vi "DereferencingPointerToComplexStructUsingGetValueByPointer.vi"(8 "error in (no error)":errorcluster, 11 "Pointer":i64) -> (0 "error out":errorcluster, 3 "ComplexStruct Polygon":T1)   [LabVIEW 2009, in "LabVIEWWrapper_PassingDataSampleDLL.lvlib"]
uses:
  LabVIEWWrapper_PassingDataSampleDLL.lvlib
  CustomControlsForStructs/ComplexStruct Polygon.ctl
  <vilib>/Utility/importsl/GetValueByPointer/GetValueByPointer.xnode
  <vilib>/Utility/importsl/GetValueByPointer/datatype.ctl
  Program Files (x86)/National Instruments/LabVIEW 2009/resource/lvimptsl.dll
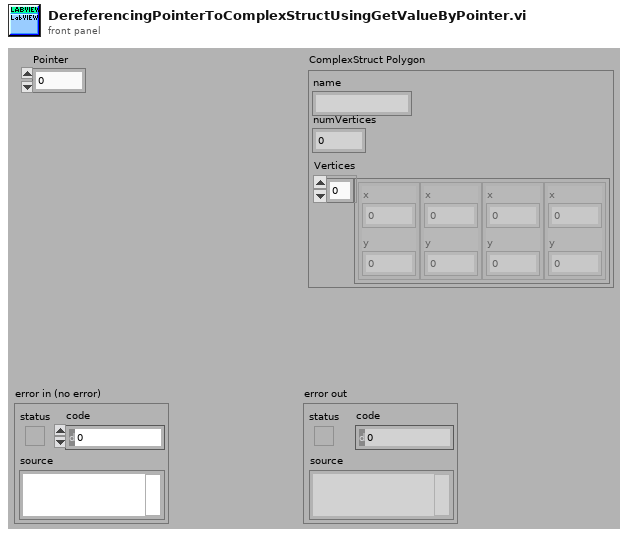
[diagram p1: front panel]
types:
  T1 = typedef "LabVIEWWrapper_PassingDataSampleDLL.lvlib/ComplexStruct Polygon.ctl" = cluster{"name":string, "numVertices":i32, "Vertices":cluster{"x":i32, "y":i32}[]}
  T2 = cluster{"Output":string, "Output":i32, cluster{"Output":i32, "Output":i32}[]}
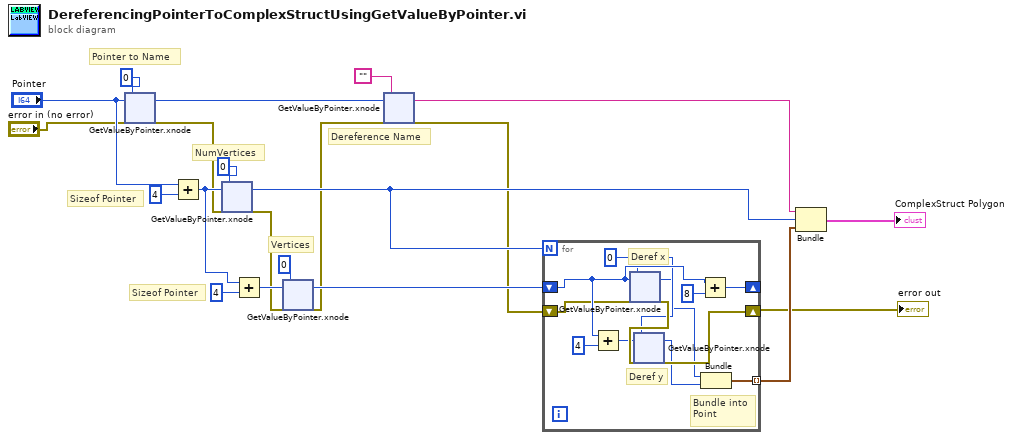
[diagram p0: block diagram]
diagram:
  # "Sizeof Pointer"
  # "Sizeof Pointer"
  # "Dereference Name"
  # "Vertices"
  # "NumVertices"
  # "Pointer to Name"
  n1 = xnode "GetValueByPointer.xnode"("Pointer"="Pointer", "InputType"=0, "ErrorIn"="error in (no error)") -> ("Output"=w20:i32, "ErrorOut"=w6:errorcluster)  [unwired: 1 in]
  n2 = Add(x="Pointer", y=i64 4) -> (x+y=w15:i64)
  n3 = xnode "GetValueByPointer.xnode"("Pointer"=w15, "InputType"=0, "ErrorIn"=w6) -> ("Output"=w9:i32, "ErrorOut"=w5:errorcluster)  [unwired: 1 in]
  n4 = Add(x=w15, y=i64 4) -> (x+y=w16:i64)
  n5 = xnode "GetValueByPointer.xnode"("Pointer"=w16, "InputType"=0, "ErrorIn"=w5) -> ("Output"=w14:i32, "ErrorOut"=w3:errorcluster)  [unwired: 1 in]
  n6 = xnode "GetValueByPointer.xnode"("Pointer"=w20, "InputType"="", "ErrorIn"=w3) -> ("Output"=w10:string, "ErrorOut"=w1:errorcluster)  [unwired: 1 in]
  n7 = for {
    N: w9 -> [_]
    shift-right: [w28] -> _
    shift-left: w14 -> [w29]
    shift-right: [w26] -> w4
    shift-left: w1 -> [w27]
    tunnel: [w22] -> w8 mode=indexing
    w25 = 0
    # "Deref y"
    # "Deref x"
    # "Bundle into\nPoint"
    n8 = Add(x=w29, y=4) -> (x+y=w32:i32)
    n9 = xnode "GetValueByPointer.xnode"("Pointer"=w29, "InputType"=w25, "ErrorIn"=w27) -> ("Output"=w24:i32, "ErrorOut"=w33:errorcluster)  [unwired: 1 in]
    n10 = xnode "GetValueByPointer.xnode"("Pointer"=w32, "InputType"=w25, "ErrorIn"=w33) -> ("Output"=w23:i32, "ErrorOut"=w26:errorcluster)  [unwired: 1 in]
    n11 = Add(x=w29, y=8) -> (x+y=w28:i32)
    n12 = Bundle("Output"=w24, "Output"=w23) -> (w22:cluster{"Output":i32, "Output":i32})  [unwired: 1 in]
  }
  "error out" <- w4
  n13 = Bundle("Output"=w10, "Output"=w9, w8) -> (→"ComplexStruct Polygon":T2)  [unwired: 1 in]
